vi "Wait for Acquisition Complete.vi"(8 "error in (no error)":errorcluster, 9 "Maximum Time (10000 ms)":i32=10000, 10 "Channel (0: Channel 1)":i32(ring) items=["Channel 1", "Channel 2"], 11 "VISA resource name":refnum<visa-resource-name>) -> (0 "error out":errorcluster, 3 "VISA resource name out":refnum<visa-resource-name>)   [LabVIEW 2020, in "Agilent B2900 Series.lvlib"]
doc: "Waits for the acquisition to finish. This VI should be called after Initiate VI and before Fetch Measurement VI.\n\n<B>Note:</B> \nUse this VI only with other low-level VIs. The high-level VIs automatically incorporate this functionality. This VI does not check the instrument status."
uses:
  Agilent B2900 Series.lvlib
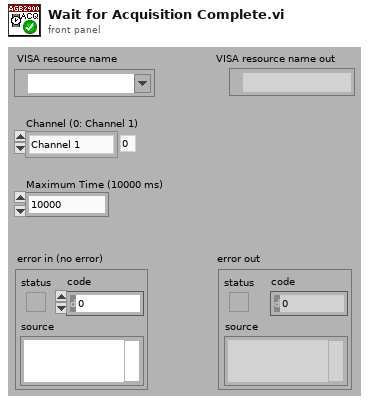
[diagram p1: front panel]
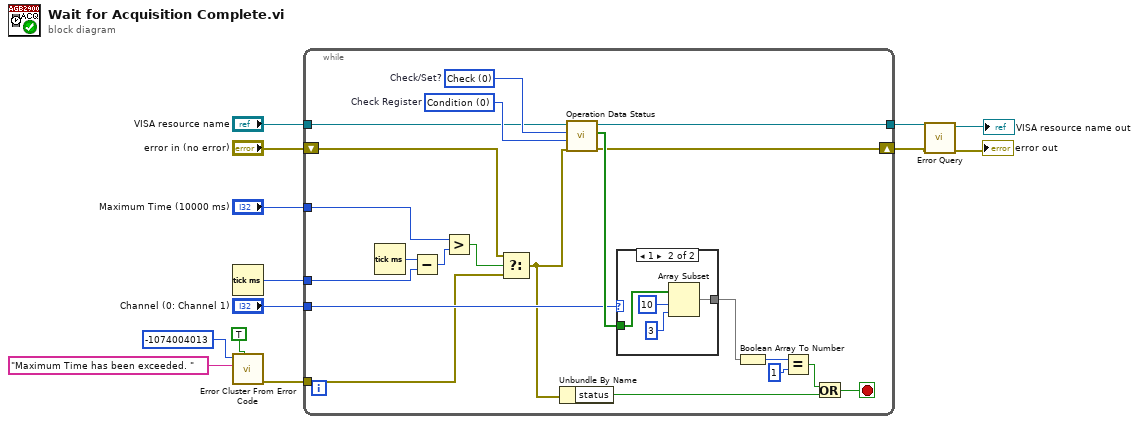
[diagram p0: block diagram]
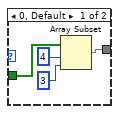
[diagram p2: hidden frame]
diagram:
  n1 = Tick Count (ms)() -> (millisecond timer value=w8:u32)
  n2 = call <vilib>:"Error Cluster From Error Code.vi"("show call chain? (False)"=TRUE, "error message (\"\")"="Maximum Time has been exceeded. " ("error message (\"\")"), "error code (0)"=-1074004013) -> ("error out"=w11:errorcluster)  [unwired: 6 in]
  n3 = while {
    tunnel: w11 -> [w22]
    tunnel: "Channel (0: Channel 1)" -> [w31]
    tunnel: w8 -> [w26]
    tunnel: "Maximum Time (10000 ms)" -> [w25]
    tunnel: "VISA resource name" -> [w21]
    shift-right: [w19] -> w3
    shift-left: "error in (no error)" -> [w23]
    tunnel: [w20] -> w4
    stop <- w18 stop-if-true
    w34 = 0 items=["Check", "Set"]  # Check/Set?
    w33 = 0 items=["Condition", "Enable", "Event", "NTR", "PTR"]  # Check Register
    n4 = Tick Count (ms)() -> (millisecond timer value=w27:u32)
    n5 = Subtract(x=w27, y=w26) -> (x-y=w24:u32)
    n6 = Greater?(x=w25, y=w24) -> (0:w16:bool)
    n7 = Select(t=w23, s=w16, f=w22) -> (s? t:f=w15:errorcluster)
    n8 = Unbundle By Name(w15) -> ("status"=w14:bool)
    n9 = call "Operation Data Status.vi"("error in (no error)"=w15, "Operation Register To Check (0: Condition)"=w33, "Operation Mode (0: Check)"=w34, "VISA resource name"=w21) -> ("error out"=w19:errorcluster, "Operation Register Status"=w32:bool[], "VISA resource name out"=w20:refnum<visa-resource-name>)  [unwired: 5 in]
    n10 = case shown="1" w31 {
      tunnel: [w36 w42] -> w30
      tunnel: w32 -> [w35 w39]
      frame 0, Default {
        n11 = Array Subset(array=w35, index=4, length=3) -> (w36:bool[])
      }
      frame 1 {
        n12 = Array Subset(array=w39, index=10, length=3) -> (w42:bool[])
      }
    }
    n13 = Boolean Array To Number(Boolean array=w30) -> (number=w29:u32)
    n14 = Equal?(x=w29, y=u32 1) -> (x = y?=w17:bool)
    n15 = Or(x=w17, y=w14) -> (x .or. y?=w18:bool)
  }
  n16 = call "Error Query.vi"("error in (no error)"=w3, "VISA resource name"=w4) -> ("error out"=→"error out":errorcluster, "VISA resource name out"=→"VISA resource name out":refnum<visa-resource-name>)  [unwired: 6 in, 2 out]
